vi "View LDA time traces.vi"() -> (5 "Plug in titles":string[](array[string]), 7 "Plug in values":string[](array[string]))   [LabVIEW 2010]
uses:
  Globals/Meas_global.vi
  Globals/Plug_in_data_global.vi
  Globals/LDA_meas_global_1.vi
panel:
  out "XY Graph":cluster{dbl[], dbl[]}[](graph)
  in  "Data Type":T1(ring)
  in  "Data to save":i32[](array[ring])=[1] items=["LDA (U)", "LDA (V)", "FF (C) Sync", "Save Nothing"]
  # "Run this VI to update the channel names"
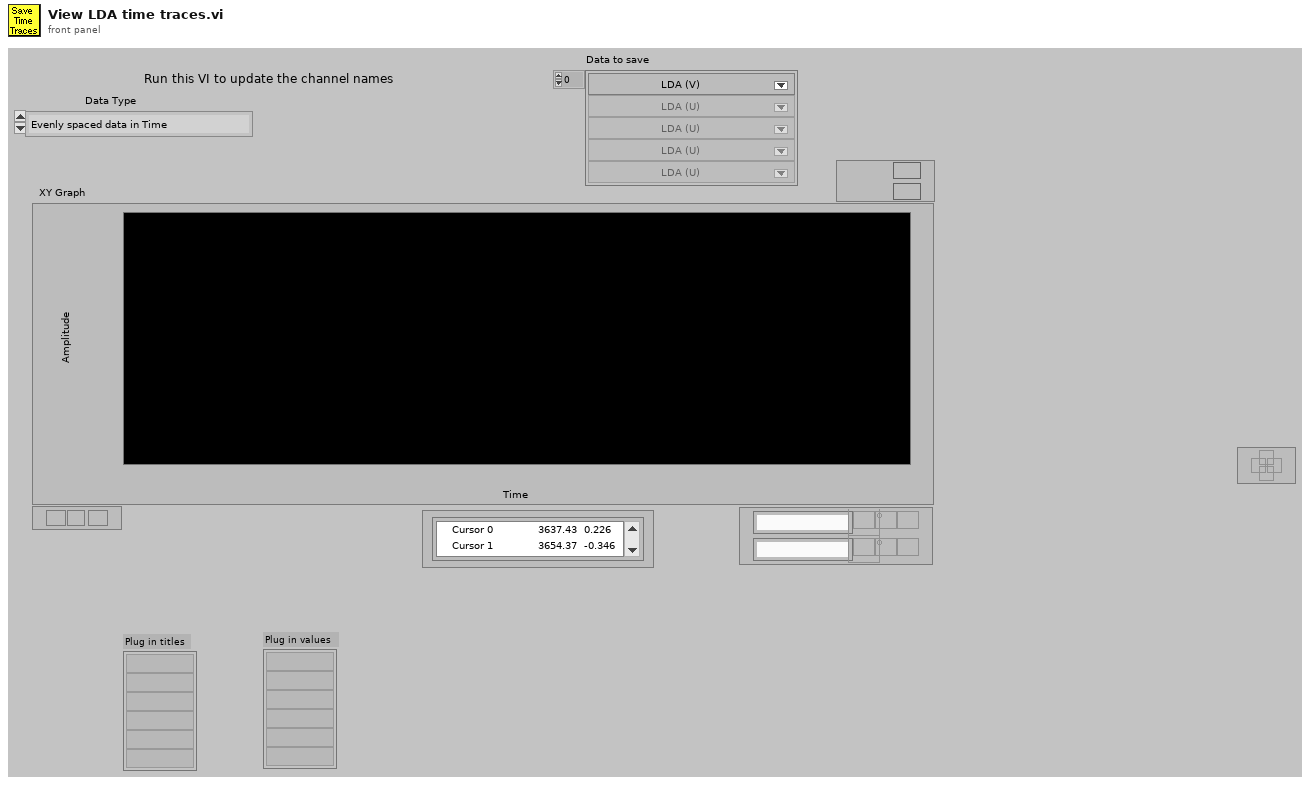
[diagram p1: front panel]
types:
  T1 = enum16{"Evenly spaced data in Time", "Unevenly spaced data in Time"}
  T2 = typedef "Analysis_info_cluster.ctl" = cluster{"Colour":u32, "Inst type":T3, "Inst name":string, "Symbol":string, "Code name":string, "Extra Info":string, "Inst Array":T4, "Index":i32, "Voltage Index":i32, "Extra Titles":string[], "Extra Values":string[]}
  T3 = typedef "Inst_type.ctl" = enum16{"Propeller anemometer", "Raw voltage", "Pressure Transducer", "Pitot-static tube", "Preston tube", "Hot wire", "Cross wire 1", "Cross wire 2", "Generic Linear", "Generic Polynomial", "Generic BackPoly", "Fast FID", "Thermocouple", "Cold wire", "Pulsed Wire", "LDA Vel", "LDA Tran time", "LDA Arr time"}
  T4 = typedef "Instrument_Array.ctl" = enum16{"PWA", "LDA", "Analogue"}
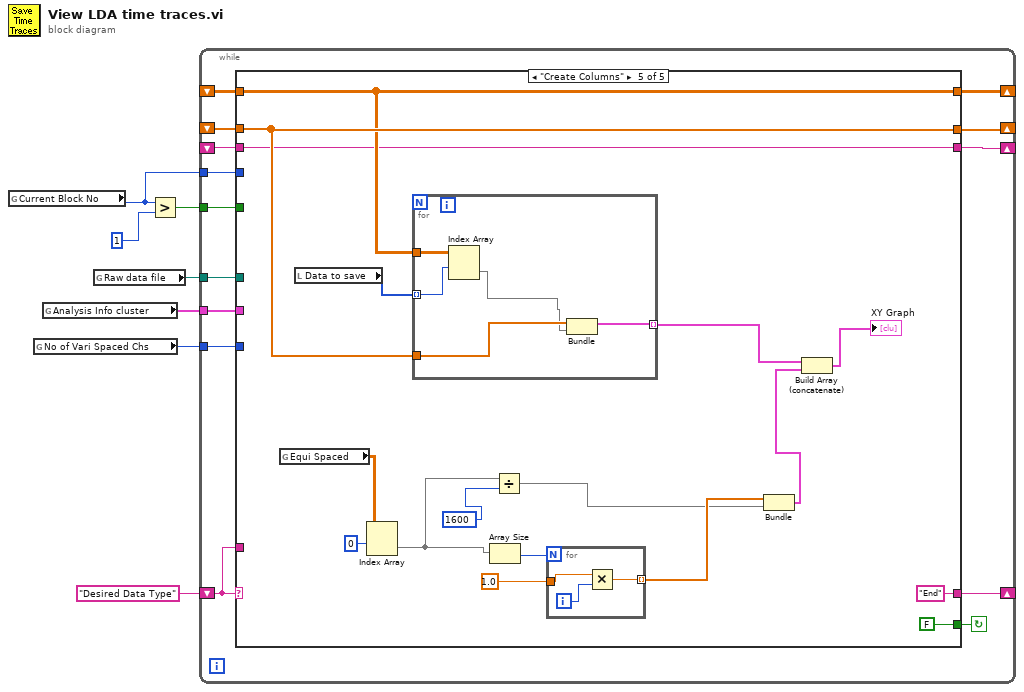
[diagram p0: block diagram]
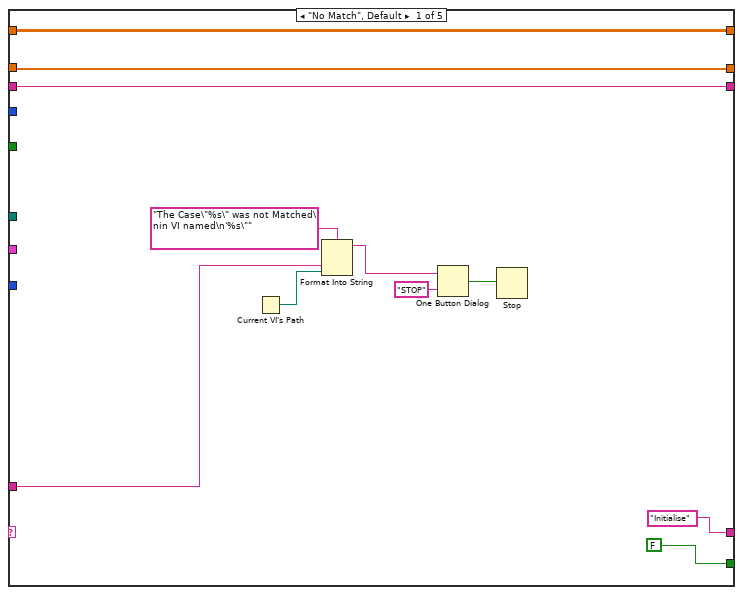
[diagram p2: hidden frame]
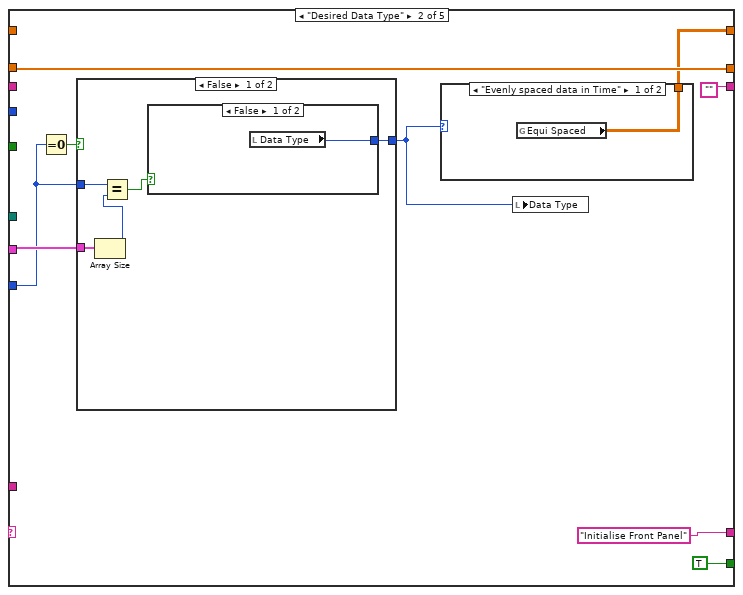
[diagram p3: hidden frame]
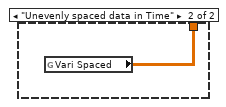
[diagram p4: hidden frame]
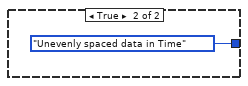
[diagram p5: hidden frame]
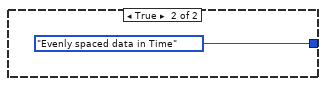
[diagram p6: hidden frame]
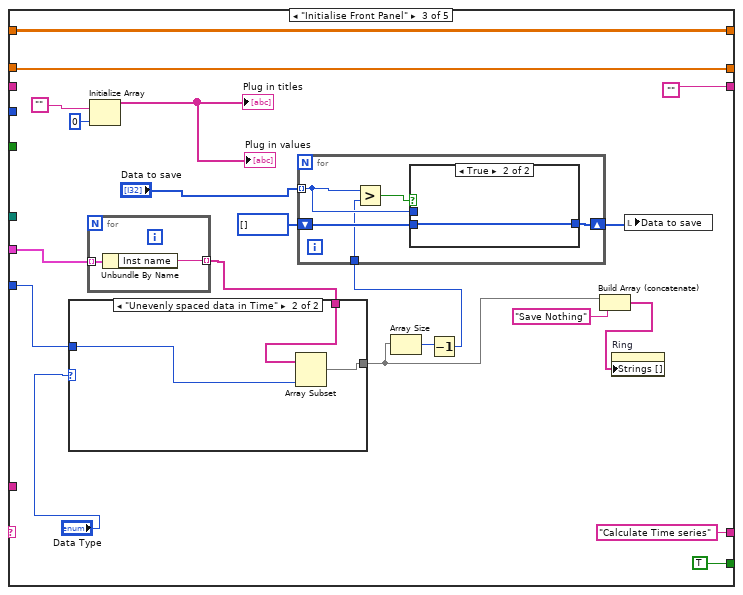
[diagram p7: hidden frame]
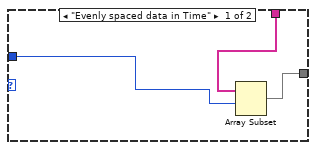
[diagram p8: hidden frame]
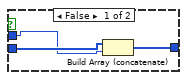
[diagram p9: hidden frame]
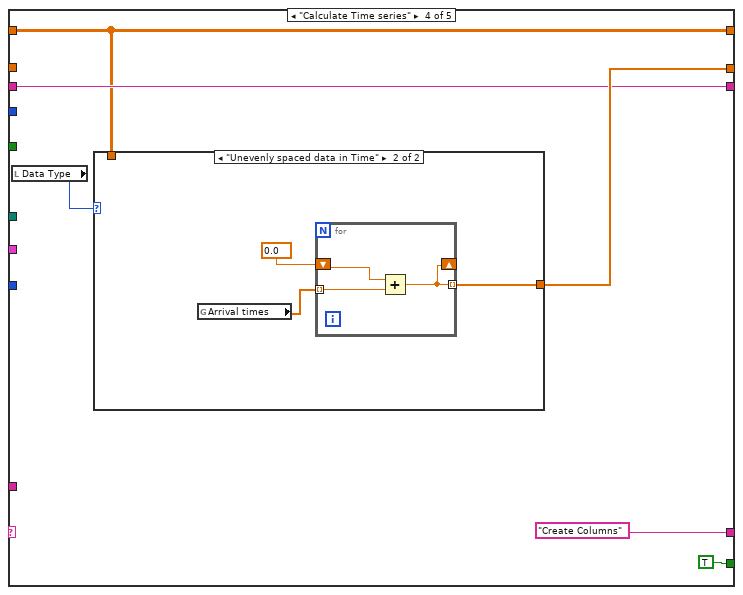
[diagram p10: hidden frame]
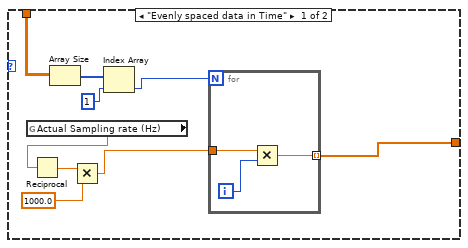
[diagram p11: hidden frame]
diagram:
  n1 = global read "Meas_global.vi" "Current Block No"() -> (w3:i32)
  n2 = global read "Meas_global.vi" "No of Vari Spaced Chs"() -> (w1:i32)
  n3 = global read "Meas_global.vi" "Analysis Info cluster"() -> (w2:T2[])
  n4 = global read "Meas_global.vi" "Raw data file"() -> (w6:path)
  n5 = Greater?(x=w3, y=1) -> (0:w4:bool)
  n6 = while {
    shift-left: "Desired Data Type" -> [w19]
    shift-right: [w20] -> _
    shift-right: [w17] -> _
    shift-left: _ -> [w16]
    tunnel: w6 -> [w18]
    tunnel: w4 -> [w15]
    shift-right: [w14] -> _
    shift-left: _ -> [w13]
    tunnel: w3 -> [w12]
    tunnel: w2 -> [w11]
    tunnel: w1 -> [w10]
    shift-right: [w9] -> _
    shift-left: _ -> [w8]
    stop <- w21 continue-if-true
    n7 = case shown="\"Create Columns\"" w19 {
      tunnel: [FALSE TRUE TRUE TRUE FALSE] -> w21
      tunnel: ["Initialise" "Initialise Front Panel" "Calculate Time series" ("t") "Create Columns" ("t") "End"] -> w20
      tunnel: w19 -> [w27 _ _ _ _]
      tunnel: w18 -> [_ _ _ _ _]
      tunnel: [w24 "" "" w91 w124] -> w17
      tunnel: w16 -> [w24 _ _ w91 w124]
      tunnel: w15 -> [_ _ _ _ _]
      tunnel: [w23 w40 w70 w93 w127] -> w14
      tunnel: w13 -> [w23 w40 w70 _ w127]
      tunnel: w12 -> [_ _ _ _ _]
      tunnel: w11 -> [_ w36 w66 _ _]
      tunnel: w10 -> [_ w35 w56 _ _]
      tunnel: [w22 w33 w55 w89 w125] -> w9
      tunnel: w8 -> [w22 _ w55 w89 w125]
      frame "No Match", Default {
        n8 = Current VI's Path() -> (path=w26:path)
        n9 = Format Into String(format string="The Case\"%s\" was not Matched\nin VI named\n'%s\"" ("Format String"), w27, w26) -> (resulting string=w30:string)  [unwired: 2 in, 1 out]
        n10 = One Button Dialog(message=w30, button name ("OK")="STOP") -> (true=w28:bool)
        n11 = Stop(stop? (T)=w28) -> ()
      }
      frame "Desired Data Type" {
        n12 = Equal To 0?(x=w35) -> (x = 0?=w39:bool)
        n13 = case shown="False" w39 {
          tunnel: [w44 T1."Evenly spaced data in Time" ("Data Type")] -> w34
          tunnel: w36 -> [w48 _]
          tunnel: w35 -> [w46 _]
          frame False {
            n14 = Array Size(array=w48) -> (size(s)=w47:i32)
            n15 = Equal?(x=w46, y=w47) -> (x = y?=w45:bool)
            n16 = case shown="False" w45 {
              tunnel: [w49 T1."Unevenly spaced data in Time" ("Data Type")] -> w44
              frame False {
                n17 = local read "Data Type"() -> (w49:T1)
              }
              frame True {
              }
            }
          }
          frame True {
          }
        }
        n18 = case shown="\"Evenly spaced data in Time\"" w34 {
          tunnel: [w42 w43] -> w33
          frame "Evenly spaced data in Time" {
            n19 = global read "Plug_in_data_global.vi" "Equi Spaced"() -> (w42:dbl[][])
          }
          frame "Unevenly spaced data in Time" {
            n20 = global read "Plug_in_data_global.vi" "Vari Spaced"() -> (w43:dbl[][])
          }
        }
        n21 = local write "Data Type"(w34) -> ()
      }
      frame "Initialise Front Panel" {
        n22 = for {
          tunnel: w66 -> [w88] mode=indexing
          tunnel: [w87] -> w60 mode=indexing
          n23 = Unbundle By Name(w88) -> ("Inst name"=w87:string)
        }
        n24 = case shown="\"Unevenly spaced data in Time\"" "Data Type" {
          tunnel: w60 -> [w74 w77]
          tunnel: [w73 w76] -> w59
          tunnel: w56 -> [w72 w75]
          frame "Evenly spaced data in Time" {
            n25 = Array Subset(array=w74, index=w72) -> (w73:string[])  [unwired: 1 in]
          }
          frame "Unevenly spaced data in Time" {
            n26 = Array Subset(array=w77, length=w75) -> (w76:string[])  [unwired: 1 in]
          }
        }
        n27 = Initialize Array("", 0) -> (→"Plug in values" →"Plug in titles":string[])
        n28 = Array Size(array=w59) -> (size(s)=w58:i32)
        n29 = Decrement(x=w58) -> (x-1=w57:i32)
        n30 = for {
          tunnel: "Data to save" -> [w79] mode=indexing
          shift-right: [w80] -> w64
          shift-left: i32[] [] -> [w81]
          tunnel: w57 -> [w78]
          n31 = Greater?(x=w79, y=w78) -> (0:w82:bool)
          n32 = case shown="True" w82 {
            tunnel: w81 -> [w85 w86]
            tunnel: [w84 w86] -> w80
            tunnel: w79 -> [w83 _]
            frame False {
              n33 = Build Array (concatenate)(w85, w83) -> (w84:i32[])
            }
            frame True {
            }
          }
        }
        n34 = Build Array (concatenate)(w59, "Save Nothing") -> (w62:string[])
        n35 = property on="Ring" class="Ring (strict)"("Strings []"=w62) -> ()  [unwired: 2 in, 2 out]
        n36 = local write "Data to save"(w64) -> ()
      }
      frame "Calculate Time series" {
        n37 = local read "Data Type"() -> (w90:T1)
        n38 = case shown="\"Unevenly spaced data in Time\"" w90 {
          tunnel: [w100 w107] -> w93
          tunnel: w89 -> [w98 _]
          frame "Evenly spaced data in Time" {
            n39 = global read "Meas_global.vi" "Actual Sampling rate (Hz)"() -> (w95:dbl)
            n40 = Reciprocal(x=w95) -> (1/x=w103:dbl)
            n41 = Array Size(array=w98) -> (size(s)=w99:i32[])
            n42 = Multiply(x=w103, y=1000.0) -> (x*y=w101:dbl)
            n43 = Index Array(array=w99, index=1) -> (element=w96:i32)
            n44 = for {
              N: w96 -> [_]
              tunnel: w101 -> [w105]
              tunnel: [w104] -> w100 mode=indexing
              i -> [w106]
              n45 = Multiply(x=w105, y=w106) -> (x*y=w104:dbl)
            }
          }
          frame "Unevenly spaced data in Time" {
            n46 = global read "LDA_meas_global_1.vi" "Arrival times"() -> (w109:dbl[])
            n47 = for {
              shift-right: [w110] -> _
              shift-left: 0.0 -> [w112]
              tunnel: w109 -> [w111] mode=indexing
              tunnel: [w110] -> w107 mode=indexing
              n48 = Add(x=w112, y=w111) -> (x+y=w110:dbl)
            }
          }
        }
      }
      frame "Create Columns" {
        n49 = global read "Plug_in_data_global.vi" "Equi Spaced"() -> (w123:dbl[][])
        n50 = local read "Data to save"() -> (w126:i32[])
        n51 = Index Array(array=w123, index (row)=0) -> (element=w117:dbl[])  [unwired: 1 in]
        n52 = for {
          tunnel: w126 -> [w136] mode=indexing
          tunnel: w125 -> [w137]
          tunnel: w127 -> [w135]
          tunnel: [w134] -> w115 mode=indexing
          n53 = Index Array(array=w137, index (row)=w136) -> (element=w133:dbl[])  [unwired: 1 in]
          n54 = Bundle(w135, "Vari Spaced"=w133) -> (w134:cluster{dbl[], "Vari Spaced":dbl[]})  [unwired: 1 out]
        }
        n55 = Array Size(array=w117) -> (size(s)=w116:i32)
        n56 = Divide(x=w117, y=1600) -> (x/y=w118:dbl[])
        n57 = for {
          N: w116 -> [_]
          tunnel: 1.0 -> [w131]
          tunnel: [w130] -> w119 mode=indexing
          i -> [w132]
          n58 = Multiply(x=w131, y=w132) -> (x*y=w130:dbl)
        }
        n59 = Bundle(w119, w118) -> (w114:cluster{dbl[], dbl[]})  [unwired: 1 out]
        n60 = Build Array (concatenate)(w115, w114) -> (→"XY Graph":cluster{dbl[], "Vari Spaced":dbl[]}[])
      }
    }
  }
